vi "Switch_Connect.vi"(8 "error in (no error)":errorcluster caption="错误输入（无错误）", 10 "COM":refnum<visa-resource-name> caption="VISA资源名称") -> (0 "error out":errorcluster, 2 "COM Out":refnum<visa-resource-name> caption="VISA资源名称输出")   [LabVIEW 2018, in "Switch.lvlib"]
uses:
  Switch.lvlib
  <vilib>/Instr/_visa.llb/VISA Configure Serial Port (Instr).vi
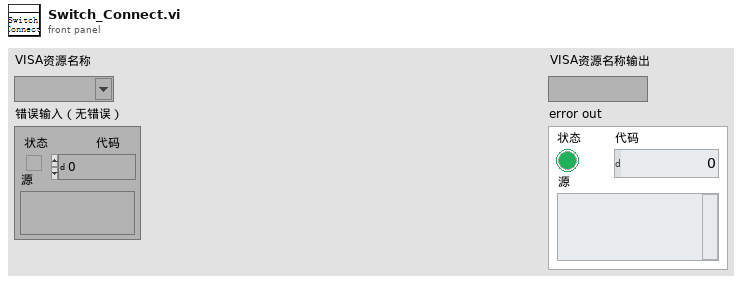
[diagram p1: front panel]
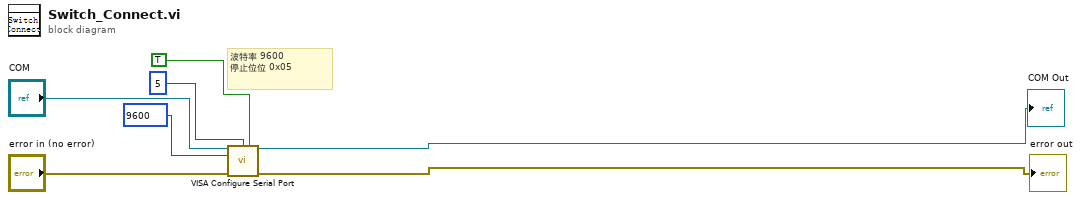
[diagram p0: block diagram]
diagram:
  # "波特率 9600\n停止位位 0x05"
  n1 = call-poly "VISA Configure Serial Port"("VISA resource name"="COM", "termination char\n(0xA = '\\n' = LF)"=u8 5 ("termination char\n(0xA = '\\n' = LF)"), "Enable Termination\nChar (T)"=TRUE ("Enable Termination\nChar (T)"), "baud rate (9600)"=u32 9600, "error in (no error)"="error in (no error)") -> ("VISA resource name out"=→"COM Out":refnum<visa-resource-name>, "error out"=→"error out":errorcluster)  [unwired: 9 in]
